vi "SaveAs.vi"(11 "PluginIniFilePath":path) -> (3 "PluginIniFilePath":path)   [LabVIEW 2018]
uses:
  <vilib>/Utility/config.llb/NI_LVConfig.lvlib
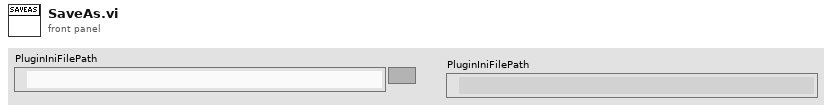
[diagram p1: front panel]
types:
  T1 = typedef "NI_LVConfig.lvlib/Config Data RefNum.ctl" = refnum<k1>
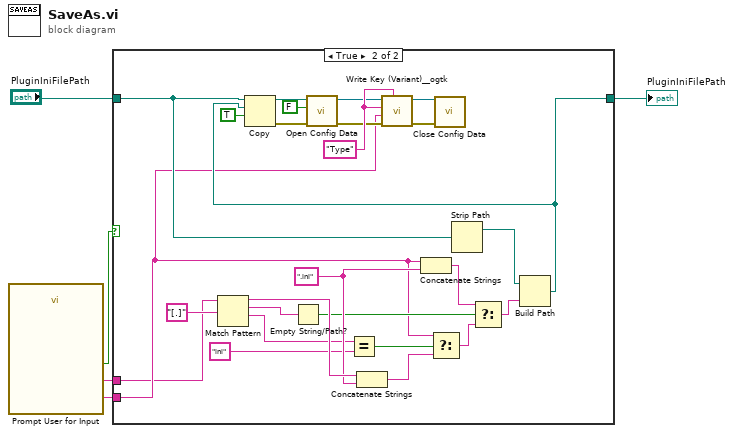
[diagram p0: block diagram]
diagram:
  n1 = call "Prompt User for Input"() -> ("Type"=w3:string, "Filename"=w2:string, "OK"=w1:bool)  [unwired: 16 in, 1 out]
  n2 = case shown="True" w1 {
    tunnel: "PluginIniFilePath" -> [w6 w10]
    tunnel: [w6 w9] -> w4
    tunnel: w3 -> [_ w8]
    tunnel: w2 -> [_ w7]
    frame False {
    }
    frame True {
      w17 = "Type" ("key (optional)")
      w30 = ".ini" ("string")
      n3 = Match Pattern(string=w7, regular expression="[.]" ("string")) -> (before substring=w31:string, match substring=w27:string, after substring=w28:string)  [unwired: 1 in, 1 out]
      n4 = Empty String/Path?(string/path=w27) -> (empty?=w22:bool)
      n5 = Equal?(x=w28, y="ini" ("string")) -> (x = y?=w24:bool)
      n6 = Concatenate Strings(w31, w30) -> (w32:string)
      n7 = Concatenate Strings(w8, w30) -> (w23:string)
      n8 = Select(t=w8, s=w24, f=w32) -> (s? t:f=w25:string)
      n9 = Strip Path(path=w10) -> (stripped path=w20:path)  [unwired: 1 out]
      n10 = Select(t=w23, s=w22, f=w25) -> (s? t:f=w21:string)
      n11 = Build Path(base path=w20, name or relative path=w21) -> (appended path=w9:path)
      n12 = Copy(9:TRUE ("overwrite (F)"), 10:w9, 11:w10) -> (0:w14:errorcluster, 3:w13:path)  [unwired: 2 in, 1 out]
      n13 = call <vilib>:"Open Config Data.vi"("error in (no error)"=w14, "create file if necessary (T)"=FALSE, "configuration file path"=w13) -> ("error out"=w15:errorcluster, "refnum"=w16:T1)  [unwired: 6 in, 1 out]
      n14 = call <userlib>:"Write Key (Variant)__ogtk.vi"("section"=w17, "error in (no error)"=w15, "key-value"=w8, "key (optional)"=w17, "refnum"=w16) -> ("error out"=w19:errorcluster, "refnum out"=w18:T1)  [unwired: 5 in]
      n15 = call <vilib>:"Close Config Data.vi"("error in (no error)"=w19, "refnum"=w18) -> ()  [unwired: 8 in, 2 out]
    }
  }
  "PluginIniFilePath" <- w4
